vi "Pause Front Panel Updates.vi"(8 "error in (no error)":errorcluster, 11 "CIF_UI in":refnum<class "CIF_UI.lvclass">) -> (0 "error out":errorcluster, 3 "CIF_UI out":refnum<class "CIF_UI.lvclass">)   [LabVIEW 2021, in "CIF_UI.lvclass"]
uses:
  CIF_UI.lvclass
  CIF_UI.lvclass/CIF_UI.ctl
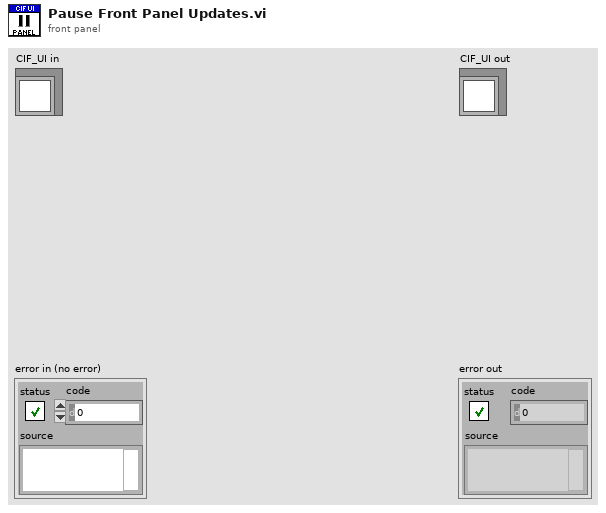
[diagram p1: front panel]
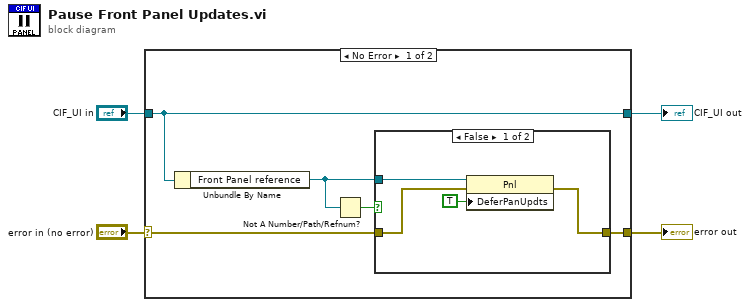
[diagram p0: block diagram]
diagram:
  n1 = case shown="No Error" "error in (no error)" {
    selector: "error in (no error)" -> [w9 w16]
    tunnel: [w6 w16] -> w3
    tunnel: [w5 w15] -> w1
    tunnel: "CIF_UI in" -> [w5 w15]
    frame No Error {
      n2 = Unbundle By Name(w5) -> ("Front Panel reference"=w8:refnum<vi>)
      n3 = Not A Number/Path/Refnum?(number/path/refnum=w8) -> (NaN/Path/Refnum?=w7:bool)
      n4 = case shown="False" w7 {
        tunnel: w9 -> [w11 w14]
        tunnel: w8 -> [w12 _]
        tunnel: [w10 w14] -> w6
        frame False {
          n5 = property class="Pnl"(reference=w12, error in=w11, "DeferPanUpdts"=TRUE ("Defer Panel Updates")) -> (error out=w10:errorcluster)  [unwired: 1 out]
        }
        frame True {
          # "FP Reference is not valid"
        }
      }
    }
    frame Error {
    }
  }
  "error out" <- w3
  "CIF_UI out" <- w1
